vi "Close.vi"(8 "error in (no error)":errorcluster, 11 "Instrument.Aerotech in":refnum<class "Instrument.Aerotech.lvclass">) -> (0 "error out":errorcluster, 3 "Instrument.Aerotech out":refnum<class "Instrument.Aerotech.lvclass">)   [LabVIEW 2019, in "Instrument.Aerotech.lvclass"]
uses:
  Instrument.Aerotech.lvclass
  <userlib>/LevyLab/Instrument Framework/Instrument Types/Delay Line/Instrument.DelayLine.lvclass
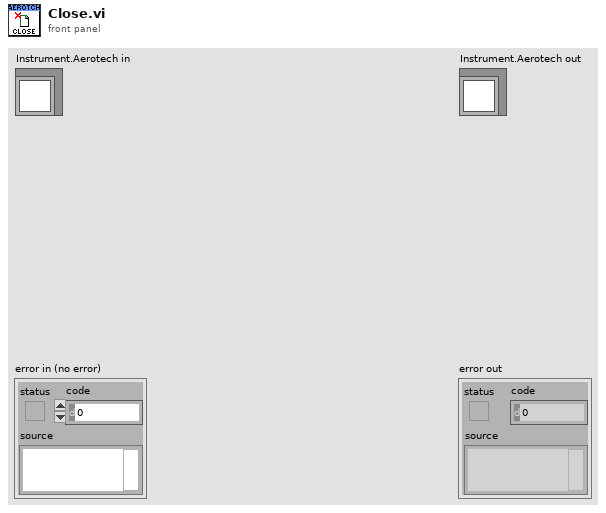
[diagram p1: front panel]
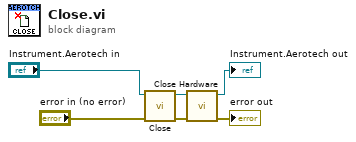
[diagram p0: block diagram]
diagram:
  n1 = call-parent "Close.vi"("error in (no error)"="error in (no error)", "Instrument in"="Instrument.Aerotech in") -> ("error out"=w2:errorcluster, "Instrument out"=w4:refnum<class "Instrument.Aerotech.lvclass">)  [unwired: 8 in]
  n2 = call-dynamic "Close Hardware.vi"("error in (no error)"=w2, "Instrument.Aerotech in"=w4) -> ("error out"=→"error out":errorcluster, "Instrument.Aerotech out"=→"Instrument.Aerotech out":refnum<class "Instrument.Aerotech.lvclass">)  [unwired: 8 in]
